vi "Actor Core.vi"(8 "error in":errorcluster, 11 "Map View in":refnum<class "Map View.lvclass">) -> (0 "error out":errorcluster, 3 "Actor out":refnum<class "Actor.lvclass">)   [LabVIEW 2020, in "Map View.lvlib" / "Map View.lvclass"]
doc: "(<B>Filename</B>: Actor Framework.lvlib:Actor.lvclass:Actor Core.vi)\n\nReceives messages to the actor, reacts to them, and initiates any error handling that may shut the actor down.\n\nDescendant classes may override this VI to append parallel tasks for the actor to complete while it handles messages. Overrides use the Call Parent Method node."
uses:
  Map View.lvclass
  C:/Program Files/National Instruments/LabVIEW 2020/vi.lib/ActorFramework/Actor/Actor.lvclass
  <vilib>/ActorFramework/Actor/Actor.lvclass
  Map View.lvclass/Map View.ctl
  <vilib>/ActorFramework/Actor/Actor.lvclass/Actor.ctl
  <vilib>/ActorFramework/Message Enqueuer/Message Enqueuer.lvclass/Message Enqueuer.ctl
  Map View Messages/Broadcast Mouse Down Msg/Broadcast Mouse Down Msg.lvclass/Broadcast Mouse Down Msg.ctl
  Map View Messages/Broadcast Mouse Move Msg/Broadcast Mouse Move Msg.lvclass/Broadcast Mouse Move Msg.ctl
  Map View Messages/Broadcast Mouse Up Msg/Broadcast Mouse Up Msg.lvclass/Broadcast Mouse Up Msg.ctl
  <vilib>/ActorFramework/Message Enqueuer/Init from Existing Queue.vi
  <vilib>/ActorFramework/Message Enqueuer/Enqueue.vi
  Map View Messages/Broadcast Mouse Down Msg/Broadcast Mouse Down Msg.lvclass
  C:/Program Files/National Instruments/LabVIEW 2020/vi.lib/ActorFramework/Message/Message.lvclass
  Map View Messages/Broadcast Mouse Move Msg/Broadcast Mouse Move Msg.lvclass
  Map View Messages/Broadcast Mouse Up Msg/Broadcast Mouse Up Msg.lvclass
  Map View Messages/Broadcast Mouse Enter Msg/Broadcast Mouse Enter Msg.lvclass
  Map View Messages/Broadcast Mouse Leave Msg/Broadcast Mouse Leave Msg.lvclass
  <vilib>/ActorFramework/Message Priority Queue/Priority Enqueue.vi
  <vilib>/ActorFrameworkMVC/Abstract View/Abstract View/Abstract View.lvclass
  <vilib>/ActorFramework/Message Enqueuer/Message Enqueuer.lvclass
panel:
  out "Grid":picture
  out "Map":picture
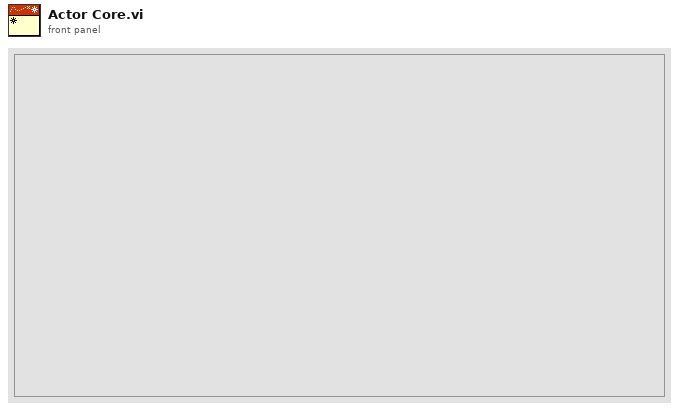
[diagram p1: front panel]
types:
  T1 = typedef "LVPoint32TypeDef.ctl" = cluster{"Horizontal":i32, "Vertical":i32}
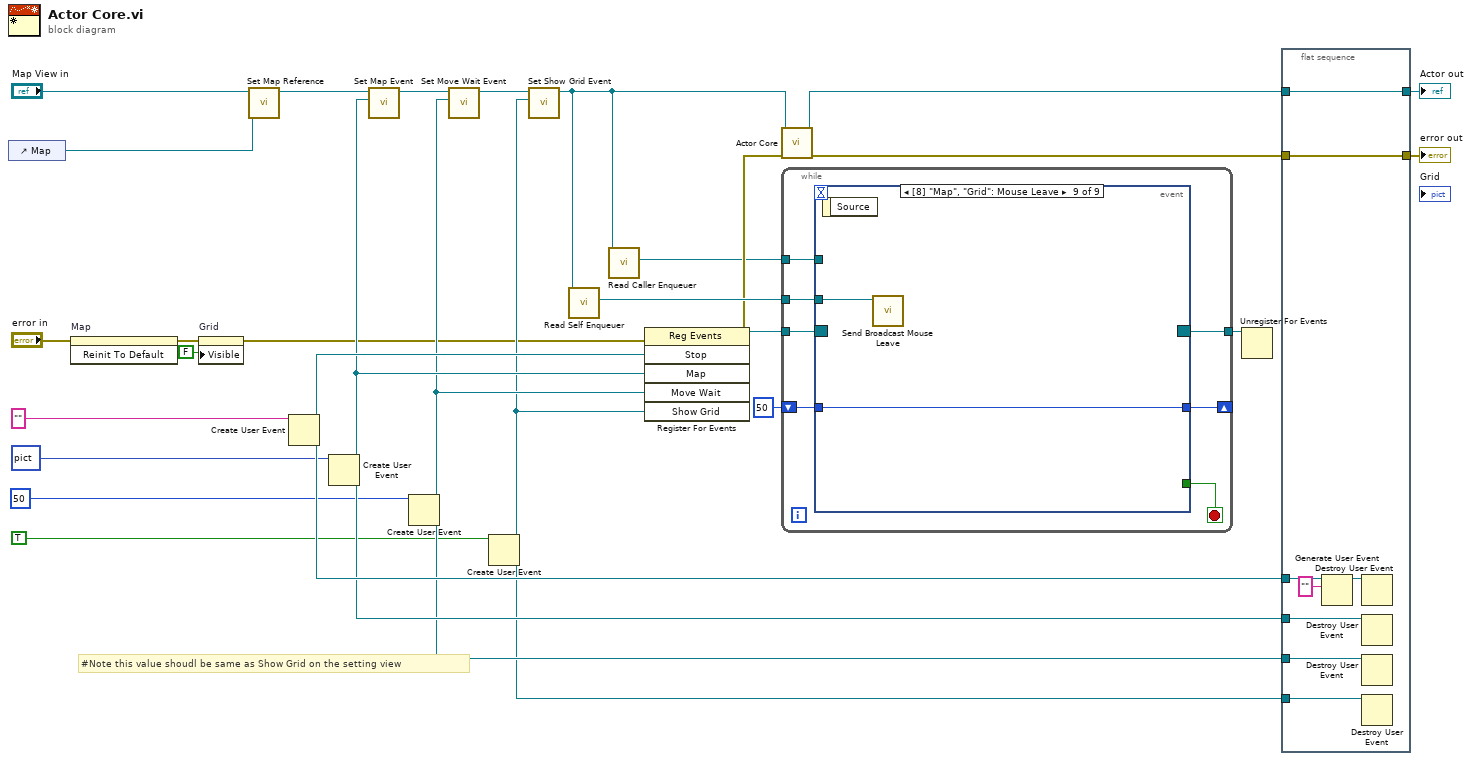
[diagram p0: block diagram]
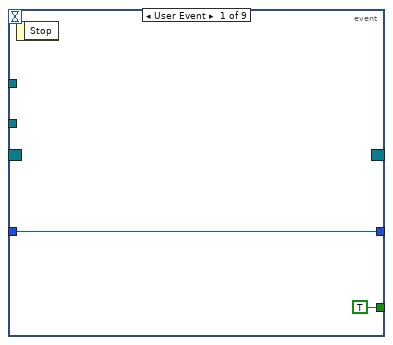
[diagram p2: hidden frame]
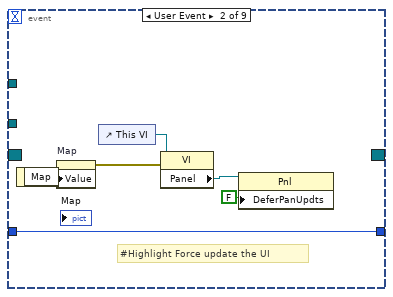
[diagram p3: hidden frame]
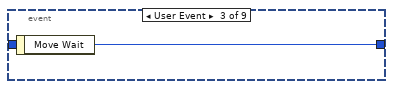
[diagram p4: hidden frame]
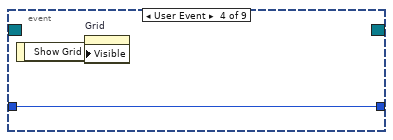
[diagram p5: hidden frame]
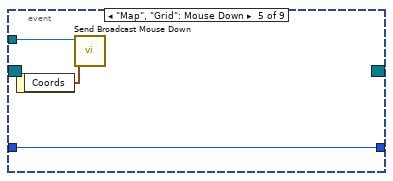
[diagram p6: hidden frame]
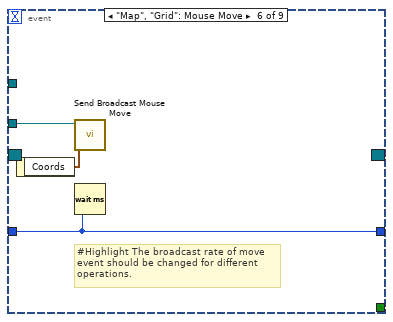
[diagram p7: hidden frame]
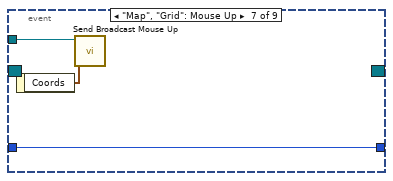
[diagram p8: hidden frame]
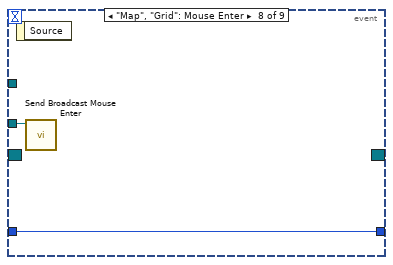
[diagram p9: hidden frame]
diagram:
  # "#Note this value shoudl be same as Show Grid on the setting view"
  n1 = control-ref of="Map"() -> (w11:refnum<vi>)
  n2 = invoke on="Map" class="Pict" method="Reinit To Default"(error in="error in") -> (error out=w3:errorcluster)  [unwired: 2 in, 2 out]
  n3 = property on="Grid" class="Pict"(error in=w3, "Visible"=FALSE) -> (error out=w2:errorcluster)  [unwired: 1 in, 1 out]
  n4 = call "Set Map Reference.vi"("Map Reference"=w11, "Map View in"="Map View in") -> ("Map View out"=w12:refnum<class "Map View.lvclass">)  [unwired: 9 in]
  n5 = Create User Event(user event datatype="" ("Stop")) -> (user event=w22:refnum<user-event>)  [unwired: 1 in, 1 out]
  n6 = Create User Event(user event datatype=picture data[5B] ("Map")) -> (user event=w16:refnum<user-event>)  [unwired: 1 in, 1 out]
  n7 = call "Set Map Event.vi"("Map Event"=w16, "Map View in"=w12) -> ("Map View out"=w14:refnum<class "Map View.lvclass">)  [unwired: 9 in]
  n8 = Create User Event(user event datatype=u32 50 ("Move Wait")) -> (user event=w7:refnum<user-event>)  [unwired: 1 in, 1 out]
  n9 = call "Set Move Wait Event.vi"("Move Wait Event"=w7, "Map View in"=w14) -> ("Map View out"=w8:refnum<class "Map View.lvclass">)  [unwired: 9 in]
  n10 = Create User Event(user event datatype=TRUE ("Show Grid")) -> (user event=w4:refnum<user-event>)  [unwired: 1 in, 1 out]
  n11 = call "Set Show Grid Event.vi"("Show Grid Event"=w4, "Map View in"=w8) -> ("Map View out"=w5:refnum<class "Map View.lvclass">)  [unwired: 9 in]
  n12 = call <vilib>:"Read Self Enqueuer.vi"("Actor"=w5) -> ("Self Enqueuer"=w23:refnum<class "Message Enqueuer.lvclass">)  [unwired: 10 in]
  n13 = call <vilib>:"Read Caller Enqueuer.vi"("Actor"=w5) -> ("Caller Enqueuer"=w13:refnum<class "Message Enqueuer.lvclass">)  [unwired: 10 in]
  n14 = register-events(error in=w2, w22, w16, w7, w4) -> (reference out=w26:refnum<event-registration>, error out=w21:errorcluster)  [unwired: 1 in]
  n15 = call-parent "Actor Core.vi"("error in"=w21, "Abstract View in"=w5) -> ("error out"=w24:errorcluster, "Actor out"=w25:refnum<class "Actor.lvclass">)  [unwired: 8 in]
  n16 = while {
    tunnel: w26 -> [w35]
    tunnel: [w34] -> w27
    tunnel: w23 -> [w32]
    tunnel: w13 -> [w31]
    shift-right: [w29] -> _
    shift-left: u32 50 -> [w30]
    stop <- w33 stop-if-true
    n17 = event shown="[8] \"Map\", \"Grid\": Mouse Leave" {
      selector: w35 -> [_ _ _ _ _ _ _ _ _]
      dyn-events: [_ _ _ _ _ _ _ _ _] -> w34
      timeout: _ -> [_ _ _ _ _ _ _ _ _]
      tunnel: [TRUE _ _ _ _ _ _ _ _] -> w33
      tunnel: w32 -> [_ _ _ _ w49 w52 w55 w56 w58]
      tunnel: w31 -> [_ _ _ _ _ _ _ _ _]
      tunnel: w30 -> [w36 w43 _ w46 w47 w50 w53 w57 w59]
      tunnel: [w36 w43 w44 w46 w47 w50 w53 w57 w59] -> w29
      event User Event {
        n18 = event-data() -> ()  [unwired: 1 in, 1 out]
      }
      event User Event {
        # "#Highlight Force update the UI"
        n19 = event-data() -> ("Map"=w39:picture)  [unwired: 1 in]
        n20 = property on="Map" class="Pict"("Value"=w39) -> (error out=w38:errorcluster)  [unwired: 2 in, 1 out]
        n21 = control-ref of="This VI"() -> (w41:refnum<vi>)
        n22 = property class="VI"(reference=w41, error in=w38) -> ("Panel"=w40:refnum<vi>)  [unwired: 2 out]
        n23 = property class="Pnl"(reference=w40, "DeferPanUpdts"=FALSE ("Defer Panel Updates")) -> ()  [unwired: 1 in, 2 out]
      }
      event User Event {
        n24 = event-data() -> ("Move Wait"=w44:u32)  [unwired: 1 in]
      }
      event User Event {
        n25 = event-data() -> ("Show Grid"=w45:bool)  [unwired: 1 in]
        n26 = property on="Grid" class="Pict"("Visible"=w45) -> ()  [unwired: 2 in, 2 out]
      }
      event "Map", "Grid": Mouse Down {
        n27 = event-data() -> ("Coords"=w48:T1)  [unwired: 1 in]
        n28 = call "Send Broadcast Mouse Down.vi"("Mouse Down"=w48, "Message Enqueuer"=w49) -> ()  [unwired: 8 in, 2 out]
      }
      event "Map", "Grid": Mouse Move {
        # "#Highlight The broadcast rate of move event should be changed for different operations."
        n29 = event-data() -> ("Coords"=w51:T1)  [unwired: 1 in]
        n30 = call "Send Broadcast Mouse Move.vi"("Mouse Move"=w51, "Message Enqueuer"=w52) -> ()  [unwired: 8 in, 2 out]
        n31 = Wait (ms)(milliseconds to wait=w50) -> ()  [unwired: 1 out]
      }
      event "Map", "Grid": Mouse Up {
        n32 = event-data() -> ("Coords"=w54:T1)  [unwired: 1 in]
        n33 = call "Send Broadcast Mouse Up.vi"("Mouse Up"=w54, "Message Enqueuer"=w55) -> ()  [unwired: 8 in, 2 out]
      }
      event "Map", "Grid": Mouse Enter {
        n34 = event-data() -> ()  [unwired: 1 in, 1 out]
        n35 = call "Send Broadcast Mouse Enter.vi"("Message Enqueuer"=w56) -> ()  [unwired: 9 in, 2 out]
      }
      event "Map", "Grid": Mouse Leave {
        n36 = event-data() -> ()  [unwired: 1 in, 1 out]
        n37 = call "Send Broadcast Mouse Leave.vi"("Message Enqueuer"=w58) -> ()  [unwired: 9 in, 2 out]
      }
    }
  }
  n38 = Unregister For Events(event registration refnum=w27) -> ()  [unwired: 1 in, 1 out]
  n39 = flat-sequence {
    tunnel: w22 -> [w66]
    tunnel: w25 -> [w64]
    tunnel: [w64] -> w19
    tunnel: [w63] -> w18
    tunnel: w24 -> [w63]
    tunnel: w16 -> [w62]
    tunnel: w7 -> [w61]
    tunnel: w4 -> [w60]
    frame #0 {
      n40 = Generate User Event(user event=w66, event data cluster="" ("event data")) -> (user event out=w67:refnum<user-event>)  [unwired: 2 in, 1 out]
      n41 = Destroy User Event(user event=w67) -> ()  [unwired: 1 in, 1 out]
      n42 = Destroy User Event(user event=w62) -> ()  [unwired: 1 in, 1 out]
      n43 = Destroy User Event(user event=w61) -> ()  [unwired: 1 in, 1 out]
      n44 = Destroy User Event(user event=w60) -> ()  [unwired: 1 in, 1 out]
    }
  }
  "error out" <- w18
  "Actor out" <- w19
